vi "FPGA Read By Name.vi"   [LabVIEW 2010, in "FPGA Interface Base.lvclass"]
doc: "Reads data from an indicator"
uses:
  <userlib>/_FPGA Interface Advanced Tools/FPGA Interface Base/FPGA Interface Base.lvclass
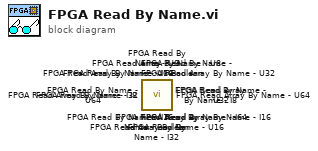
[diagram p0: block diagram]
diagram:
  n1 = call <userlib>:"FPGA Read Array By Name - Boolean.vi"() -> ()  [unwired: 9 in, 3 out]
  n2 = call <userlib>:"FPGA Read By Name - Boolean.vi"() -> ()  [unwired: 9 in, 3 out]
  n3 = call <userlib>:"FPGA Read By Name - U64.vi"() -> ()  [unwired: 9 in, 3 out]
  n4 = call <userlib>:"FPGA Read By Name - U32.vi"() -> ()  [unwired: 9 in, 3 out]
  n5 = call <userlib>:"FPGA Read By Name - U16.vi"() -> ()  [unwired: 9 in, 3 out]
  n6 = call <userlib>:"FPGA Read By Name - U8.vi"() -> ()  [unwired: 9 in, 3 out]
  n7 = call <userlib>:"FPGA Read By Name - I64.vi"() -> ()  [unwired: 9 in, 3 out]
  n8 = call <userlib>:"FPGA Read By Name - I32.vi"() -> ()  [unwired: 9 in, 3 out]
  n9 = call <userlib>:"FPGA Read By Name - I16.vi"() -> ()  [unwired: 9 in, 3 out]
  n10 = call <userlib>:"FPGA Read By Name - I8.vi"() -> ()  [unwired: 9 in, 3 out]
  n11 = call <userlib>:"FPGA Read Array By Name - U64.vi"() -> ()  [unwired: 9 in, 3 out]
  n12 = call <userlib>:"FPGA Read Array By Name - U32.vi"() -> ()  [unwired: 9 in, 3 out]
  n13 = call <userlib>:"FPGA Read Array By Name - U16.vi"() -> ()  [unwired: 9 in, 3 out]
  n14 = call <userlib>:"FPGA Read Array By Name - U8.vi"() -> ()  [unwired: 9 in, 3 out]
  n15 = call <userlib>:"FPGA Read Array By Name - I64.vi"() -> ()  [unwired: 9 in, 3 out]
  n16 = call <userlib>:"FPGA Read Array By Name - I32.vi"() -> ()  [unwired: 9 in, 3 out]
  n17 = call <userlib>:"FPGA Read Array By Name - I16.vi"() -> ()  [unwired: 9 in, 3 out]
  n18 = call <userlib>:"FPGA Read Array By Name - I8.vi"() -> ()  [unwired: 9 in, 3 out]
